vi "Stop.vi"(8 "error in (no error)":errorcluster, 11 "Sound Visualizer in":refnum<class "Sound Visualizer.lvclass">) -> (0 "error out":errorcluster, 3 "Sound Visualizer out":refnum<class "Sound Visualizer.lvclass">)   [LabVIEW 2010, in "Sound Visualizer.lvclass"]
doc: "Stops any sound playing on the visualizer.\n\nThis method is not actually used in the Sound Demo application, but it is included for completeness and future expansion."
uses:
  Sound Visualizer.lvclass
  Sound Visualizer.lvclass/Sound Visualizer.ctl
  Visualizer/Visualizer.lvlib
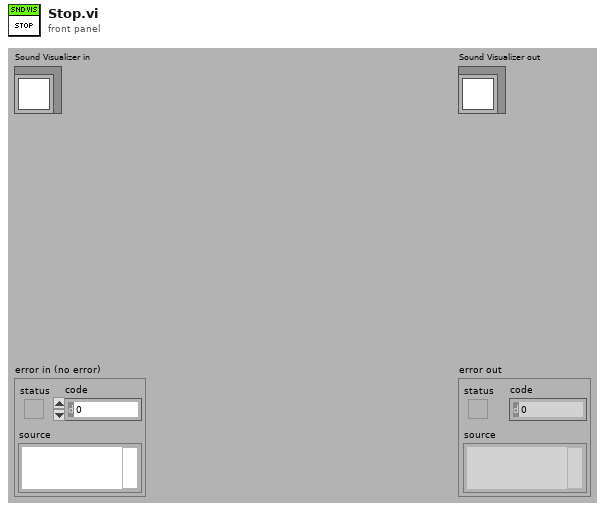
[diagram p1: front panel]
types:
  T1 = typedef "Visualizer.lvlib/Visualizer Type ID.ctl" = u32
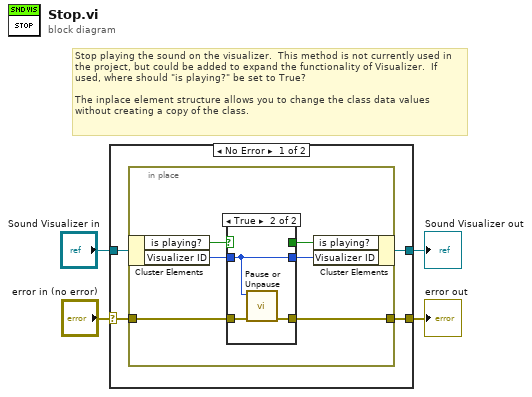
[diagram p0: block diagram]
diagram:
  # "Stop playing the sound on the visualizer.  This method is not currently used in the project, but could be added to expand the functionality of Visualizer.  If used, where should \"is playing?\" be set to True?\n\nThe inplace element structure allows you to change the class data values without creating a copy of the class."
  n1 = case shown="No Error" "error in (no error)" {
    selector: "error in (no error)" -> [w6 w22]
    tunnel: [w5 w22] -> w3
    tunnel: [w7 w21] -> w2
    tunnel: "Sound Visualizer in" -> [w8 w21]
    frame No Error {
      n2 = in-place {
        in-place-border: w6 -> [w11]
        in-place-border: [w10] -> w5
        n3 = in-place-cluster #1(w8) -> ("is playing?"=w14:bool, "Visualizer ID"=w12:T1)
        n4 = case shown="True" w14 {
          selector: w14 -> [w16 _]
          tunnel: [w16 _] -> w13
          tunnel: w12 -> [w17 w19]
          tunnel: w11 -> [w15 w20]
          tunnel: [w15 w18] -> w10
          tunnel: [w17 w19] -> w9
          frame False {
          }
          frame True {
            n5 = call "Pause or Unpause.vi"("error in (no error)"=w20, "Visualizer ID"=w19) -> ("error out"=w18:errorcluster)  [unwired: 9 in]
          }
        }
        n6 = in-place-cluster #1("is playing?"=w13, "Visualizer ID"=w9) -> (w7:refnum<class "Sound Visualizer.lvclass">)
      }
    }
    frame Error {
    }
  }
  "error out" <- w3
  "Sound Visualizer out" <- w2
